vi "Format InstancePrivateIpAddressSetItemType_LVXML_Loop.vi"(8 "error in (no error)":errorcluster, 10 "Siblings in 4":T2(array[cluster]), 11 "AWS_EC2 in":refnum<class "AWS_EC2.lvclass">) -> (0 "error out":errorcluster, 2 "Array":T3[](array[typedef]), 3 "AWS_EC2 out":refnum<class "AWS_EC2.lvclass">)   [LabVIEW 2014, in "AWS_EC2.lvlib" / "AWS_EC2.lvclass"]
uses:
  AWS_EC2.lvclass
  EC2 Datatypes/InstancePrivateIpAddressesSetItemType.ctl
  EC2 Datatypes/InstanceNetworkInterfaceAssociationType.ctl
  lv-xml-parser/r0/trunk/VI Source/EventType.ctl
  AWS_EC2.lvlib
  lv-xml-parser/r0/trunk/VI Source/LV XML Parser.lvlib
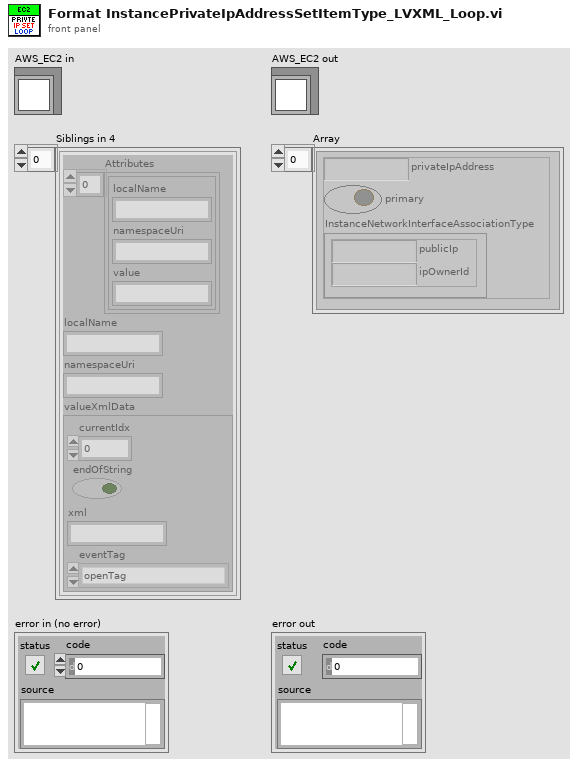
[diagram p1: front panel]
types:
  T1 = typedef "LV XML Parser.lvlib/EventType.ctl" = enum16{"openTag", "endOpenTag", "closeTag", "comment", "endComment", "endOfFile", "attribute", "startXml"}
  T2 = cluster{"Attributes":cluster{"localName":string, "namespaceUri":string, "value":string}[], "localName":string, "namespaceUri":string, "valueXmlData":cluster{"currentIdx":i32, "endOfString":bool, "xml":string, "eventTag":T1}}[]
  T3 = typedef "AWS_EC2.lvlib/InstancePrivateIpAddressesSetItemType.ctl" = cluster{"privateIpAddress":string, "primary":bool, "InstanceNetworkInterfaceAssociationType":T4}
  T4 = typedef "AWS_EC2.lvlib/InstanceNetworkInterfaceAssociationType.ctl" = cluster{"publicIp":string, "ipOwnerId":string}
  T5 = cluster{"Attributes":cluster{"localName":string, "namespaceUri":string, "value":string}[], "localName":string, "namespaceUri":string, "valueXmlData":cluster{"currentIdx":i32, "endOfString":bool, "xml":string, "eventTag":T1}}
  T6 = cluster{"currentIdx":i32, "endOfString":bool, "xml":string, "eventTag":T1}
  T7 = cluster{"namespaceUri":string, "localName":string}
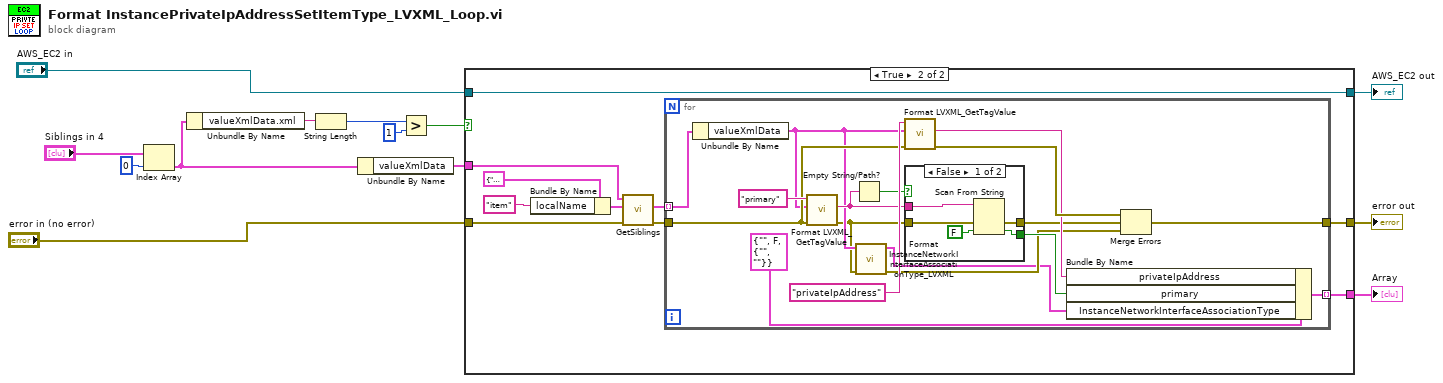
[diagram p0: block diagram]
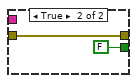
[diagram p3: hidden frame]
diagram:
  n1 = Index Array(array="Siblings in 4", index=0) -> (element=w10:T5)
  n2 = Unbundle By Name(w10) -> ("valueXmlData.xml"=w9:string)
  n3 = String Length(string=w9) -> (length=w5:i32)
  n4 = Unbundle By Name(w10) -> ("valueXmlData"=w8:T6)
  n5 = Greater?(x=w5, y=1) -> (0:w7:bool)
  n6 = case shown="True" w7 {
    tunnel: [w15 w24] -> w1
    tunnel: "error in (no error)" -> [w15 w19]
    tunnel: w8 -> [_ w18]
    tunnel: "AWS_EC2 in" -> [w14 w17]
    tunnel: [w14 w17] -> w12
    tunnel: [_ w16] -> w13
    frame False {
    }
    frame True {
      n7 = Bundle By Name(cluster=T7 {"namespaceUri"="", "localName"=""} ("limitToTag"), "localName"="item" ("Tag name")) -> (w21:T7)
      n8 = call "GetSiblings.vi"("error in (no error)"=w19, "limitToTag"=w21, "xmlData"=w18) -> ("error out"=w25:errorcluster, "Siblings"=w22:T2)  [unwired: 7 in]
      n9 = for {
        tunnel: w22 -> [w42] mode=indexing
        tunnel: [w41] -> w24
        tunnel: w25 -> [w31]
        tunnel: [w37] -> w16 mode=indexing
        n10 = Unbundle By Name(w42) -> ("valueXmlData"=w29:T6)
        n11 = call "Format LVXML_GetTagValue.vi"("error in (no error)"=w31, "xmlDataIn"=w29, "Tag name"="primary") -> ("error out"=w28:errorcluster, "Value"=w32:string)  [unwired: 6 in, 1 out]
        n12 = Empty String/Path?(string/path=w32) -> (empty?=w34:bool)
        n13 = call "Format InstanceNetworkInterfaceAssociationType_LVXML.vi"("error in (no error)"=w28, "xmlData in"=w29) -> ("error out"=w27:errorcluster, "InstanceNetworkInterfaceAssociationType"=w26:T4)  [unwired: 8 in]
        n14 = call "Format LVXML_GetTagValue.vi"("error in (no error)"=w31, "xmlDataIn"=w29, "Tag name"="privateIpAddress") -> ("error out"=w38:errorcluster, "Value"=w35:string)  [unwired: 6 in, 1 out]
        n15 = case shown="False" w34 {
          tunnel: [w47 w49] -> w30
          tunnel: [w46 FALSE] -> w33
          tunnel: w28 -> [w44 w49]
          tunnel: w32 -> [w43 _]
          frame False {
            n16 = Scan From String(input string=w43, error in=w44, default 1=FALSE) -> (error out=w47:errorcluster, output 1=w46:bool)  [unwired: 2 in, 2 out]
          }
          frame True {
          }
        }
        n17 = Bundle By Name(cluster=T3 {"privateIpAddress"="", "primary"=FALSE, "InstanceNetworkInterfaceAssociationType"={"publicIp"="", "ipOwnerId"=""}} ("InstancePrivateIpAddressesSetItemType"), "privateIpAddress"=w35, "primary"=w33, "InstanceNetworkInterfaceAssociationType"=w26) -> (w37:T3)
        n18 = Merge Errors(w38, w30, w27) -> (w41:errorcluster)
      }
    }
  }
  "Array" <- w13
  "AWS_EC2 out" <- w12
  "error out" <- w1
